vi "Exchange_Dot_Status_for_Candidates(Unmov)-1.vi"(4 "i+j":i32, 5 "Gap closed!!!":bool, 6 "Index of \ncandidate dot\ninside the frame":i32, 7 "Gap Potentially \nClosed":bool, 8 "Count of potentially\ngaps between dots":i32, 9 "previous dot\n# frame":i32, 10 "previous dot\nindex in column":i32, 11 "[IN] Dot matrix with zero \ndeleted dots":i16[][](array[numeric])) -> (3 "[OUT] Dot matrix with zero \ndeleted dots":i16[][](array[numeric]))   [LabVIEW 2017]
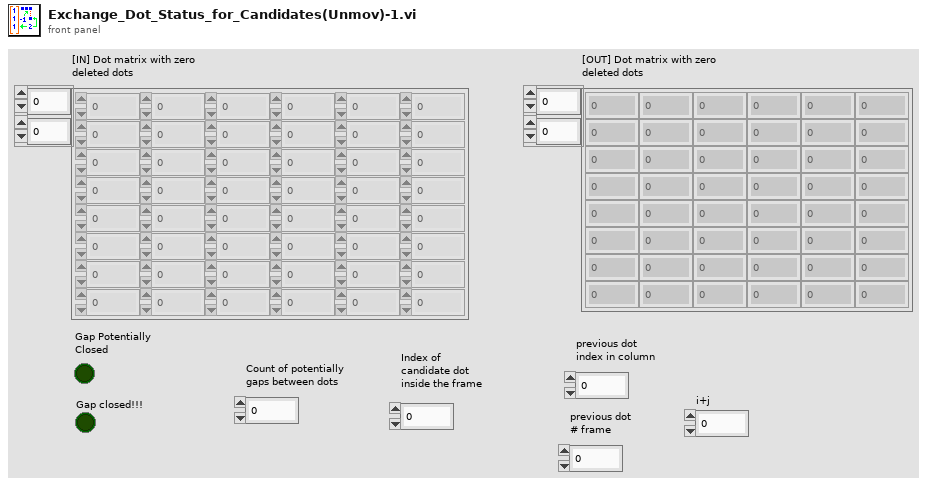
[diagram p1: front panel]
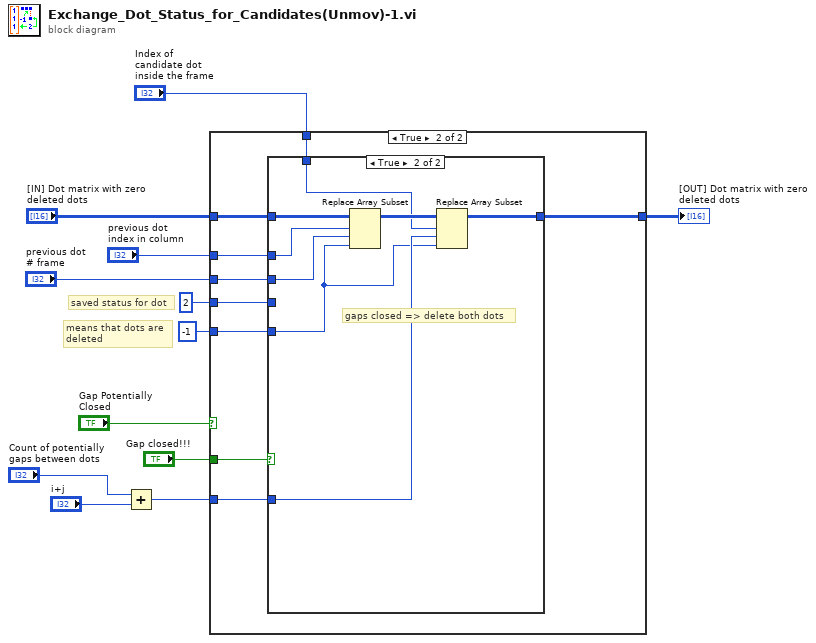
[diagram p0: block diagram]
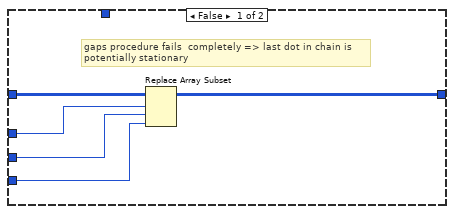
[diagram p2: hidden frame]
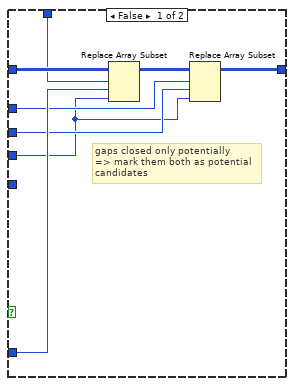
[diagram p3: hidden frame]
diagram:
  # "means that dots are \ndeleted"
  # "saved status for dot"
  n1 = Add(x="Count of potentially\ngaps between dots", y="i+j") -> (x+y=w3:i32)
  n2 = case shown="True" "Gap Potentially \nClosed" {
    tunnel: "[IN] Dot matrix with zero \ndeleted dots" -> [w17 w25]
    tunnel: "previous dot\nindex in column" -> [w15 w19]
    tunnel: "previous dot\n# frame" -> [w16 w20]
    tunnel: i16 2 -> [w14 w21]
    tunnel: [w13 w24] -> w6
    tunnel: "Gap closed!!!" -> [_ w26]
    tunnel: w3 -> [_ w23]
    tunnel: "Index of \ncandidate dot\ninside the frame" -> [_ w22]
    tunnel: i16 -1 -> [_ w18]
    frame False {
      # "gaps procedure fails  completely => last dot in chain is \npotentially stationary"
      n3 = Replace Array Subset(array=w17, new element=w14, index (row)=w15, index (col)=w16) -> (w13:i16[][])
    }
    frame True {
      n4 = case shown="True" w26 {
        tunnel: w25 -> [w34 w42]
        tunnel: [w27 w37] -> w24
        tunnel: w23 -> [w33 w38]
        tunnel: w22 -> [w31 w36]
        tunnel: w21 -> [w28 _]
        tunnel: w20 -> [w29 w41]
        tunnel: w19 -> [w30 w40]
        tunnel: w18 -> [_ w35]
        frame False {
          # "gaps closed only potentially\n=> mark them both as potential\ncandidates"
          n5 = Replace Array Subset(array=w34, new element=w28, index (row)=w31, index (col)=w33) -> (w32:i16[][])
          n6 = Replace Array Subset(array=w32, new element=w28, index (row)=w30, index (col)=w29) -> (w27:i16[][])
        }
        frame True {
          # "gaps closed => delete both dots"
          n7 = Replace Array Subset(array=w42, new element=w35, index (row)=w40, index (col)=w41) -> (w39:i16[][])
          n8 = Replace Array Subset(array=w39, new element=w35, index (row)=w36, index (col)=w38) -> (w37:i16[][])
        }
      }
    }
  }
  "[OUT] Dot matrix with zero \ndeleted dots" <- w6
